vi "数值转换.vi"(8 "error in (no error)":errorcluster caption="错误输入（无错误）", 11 "Digital Waveform":digitalwaveform(waveform)) -> (0 "error out":errorcluster caption="错误输出", 3 "Waveform":waveform(dbl))   [LabVIEW 2019]
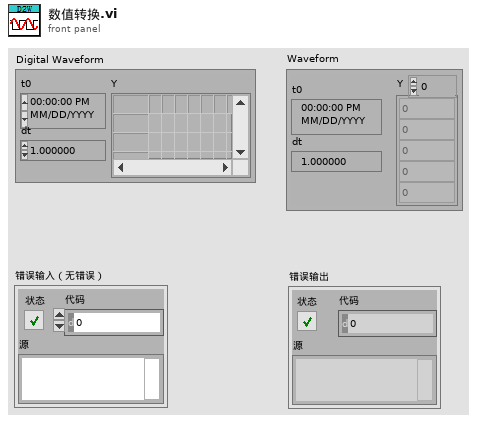
[diagram p1: front panel]
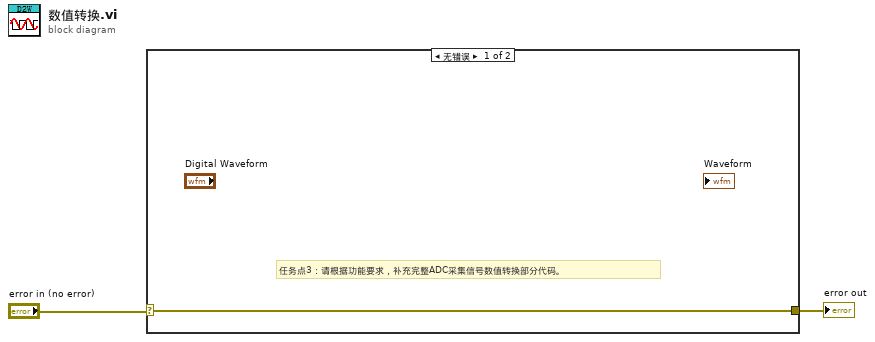
[diagram p0: block diagram]
diagram:
  n1 = case shown="无错误" "error in (no error)" {
    selector: "error in (no error)" -> [w3 w4]
    tunnel: [w3 w4] -> w1
    frame No Error {
      # "任务点3：请根据功能要求，补充完整ADC采集信号数值转换部分代码。"
    }
    frame Error {
    }
  }
  "error out" <- w1
